vi "Read WS Server ini param.vi"(8 "error in (no error)":errorcluster, 9 "configuration file path":path, 11 "WS in":T1={"WS Port"=6123, "connect timeout"=10000, "read operation timeout"=15000, "write operation timeout"=15000}) -> (0 "error out":errorcluster, 3 "WS out":T1={"WS Port"=6123, "connect timeout"=10000, "read operation timeout"=15000, "write operation timeout"=15000})   [LabVIEW 2021, in "WebSockets.lvlib" / "WebSocket Server.lvclass"]
uses:
  WebSocket Server.lvclass
  <vilib>/Utility/config.llb/Read Key (I32).vi
  <vilib>/Utility/config.llb/Read Key (U32).vi
  <vilib>/Utility/config.llb/NI_LVConfig.lvlib
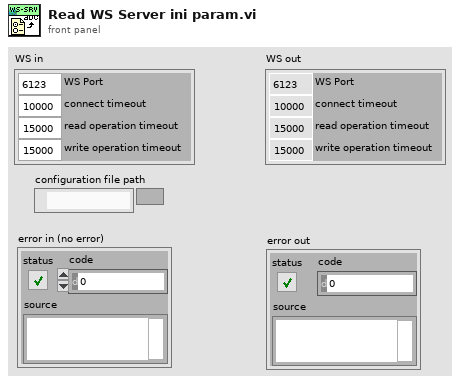
[diagram p1: front panel]
types:
  T1 = cluster{"WS Port":u16, "connect timeout":i32, "read operation timeout":i32, "write operation timeout":i32}
  T2 = typedef "NI_LVConfig.lvlib/Config Data RefNum.ctl" = refnum<k1>
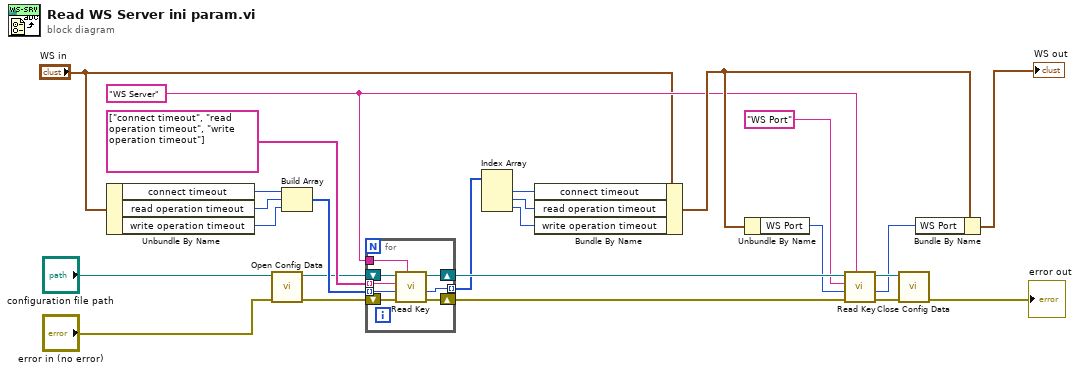
[diagram p0: block diagram]
diagram:
  w9 = "WS Server" ("key")
  n1 = Unbundle By Name("WS in") -> ("connect timeout"=w12:i32, "read operation timeout"=w11:i32, "write operation timeout"=w10:i32)
  n2 = call <vilib>:"Open Config Data.vi"("error in (no error)"="error in (no error)", "configuration file path"="configuration file path") -> ("error out"=w22:errorcluster, "refnum"=w21:T2)  [unwired: 7 in, 1 out]
  n3 = Build Array(w12, w11, w10) -> (w25:i32[])
  n4 = for {
    tunnel: w9 -> [w30]
    tunnel: w25 -> [w28] mode=indexing
    shift-right: [w27] -> w4
    shift-left: w22 -> [w33]
    shift-right: [w26] -> w19
    shift-left: w21 -> [w32]
    tunnel: string[] ["connect timeout", "read operation timeout", "write operation timeout"] -> [w31] mode=indexing
    tunnel: [w29] -> w16 mode=indexing
    n5 = call-poly <vilib>:"Read Key.vi"("section"=w30, "error in (no error)"=w33, "default value"=w28, "key"=w31, "refnum"=w32) -> ("error out"=w27:errorcluster, "value"=w29:i32, "refnum out"=w26:T2)  [unwired: 3 in, 1 out]
  }
  n6 = Index Array(array=w16) -> (element #1=w15:i32, element #2=w14:i32, element #3=w7:i32)  [unwired: 3 in]
  n7 = Bundle By Name(cluster="WS in", "connect timeout"=w15, "read operation timeout"=w14, "write operation timeout"=w7) -> (w13:T1)
  n8 = Unbundle By Name(w13) -> ("WS Port"=w5:u16)
  n9 = call-poly <vilib>:"Read Key.vi"("section"=w9, "error in (no error)"=w4, "default value"=w5, "key"="WS Port", "refnum"=w19) -> ("error out"=w3:errorcluster, "value"=w2:u32, "refnum out"=w18:T2)  [unwired: 4 out]
  n10 = call <vilib>:"Close Config Data.vi"("error in (no error)"=w3, "refnum"=w18) -> ("error out"=→"error out":errorcluster)  [unwired: 8 in, 1 out]
  n11 = Bundle By Name(cluster=w13, "WS Port"=w2) -> (→"WS out":T1)
